vi "Begin.vi"(8 "error in":errorcluster) -> (0 "error out":errorcluster)   [LabVIEW 2014]
doc: "Called before other user functions, this VI is expected to open initial I/O refnums, load in file data, and do all program initialization. Notice that the <B>error out</B> terminal is simply used for data flow. Wiring it to other structures or subVIs ensures that this VI runs first."
uses:
  <vilib>/Rock Robotics/WPI/SafetyOutput/WPI_SafetyOutputConfigMenu.ctl
  <vilib>/Rock Robotics/WPI/DriverStation/WPI_DriverStationRobotMode2.ctl
  <vilib>/Rock Robotics/WPI/Joystick/WPI_JoystickDeviceEnum.ctl
  <vilib>/Rock Robotics/SystemInterfaces/DIO/FPGA_DIOPWMChannel.ctl
  <vilib>/Rock Robotics/SystemInterfaces/spilib/spi_bus.ctl
  <vilib>/Rock Robotics/SystemInterfaces/AI/FPGA_AIGyroChannel.ctl
  <vilib>/Rock Robotics/SystemInterfaces/DIO/FPGA_DIOChannel.ctl
  <vilib>/Rock Robotics/WPI/Encoder/WPI_EncoderType.ctl
  <vilib>/Rock Robotics/WPI/Solenoid/WPI_SolenoidChannel.ctl
  Robot Global Data.vi
  <vilib>/Rock Robotics/Network Tables/SD Write String Array.vi
  <vilib>/Rock Robotics/WPI/RobotDrive/WPI_RobotDriveOpen4MotorWithTalon.vi
  <vilib>/Rock Robotics/WPI/MotorControl/WPI_MotorControlOpen Talon.vi
  <vilib>/Rock Robotics/WPI/Counter/WPI_CounterDigitalInputToDigitalSource.vi
  <vilib>/Rock Robotics/WPI/Compressor/WPI_CompressorGetSetRefNum.vi
  <vilib>/Rock Robotics/WPI/Solenoid/WPI_SolenoidOpenDouble.vi
  NavX/navX-MXP Library/navX-MXP IMU.lvlib
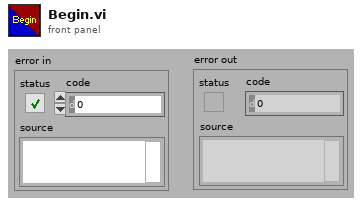
[diagram p1: front panel]
types:
  T1 = typedef "WPI_SolenoidChannel.ctl" = enum8{"Solenoid 0", "Solenoid 1", "Solenoid 2", "Solenoid 3", "Solenoid 4", "Solenoid 5", "Solenoid 6", "Solenoid 7", "Invalid"}
  T2 = typedef "WPI_JoystickDeviceEnum.ctl" = enum16{"USB 0", "USB 1", "USB 2", "USB 3", "USB 4", "USB 5"}
  T3 = typedef "WPI_EncoderType.ctl" = enum16{"1x", "2x", "4x"}
  T4 = typedef "FPGA_DIOPWMChannel.ctl" = enum8{"PWM 0", "PWM 1", "PWM 2", "PWM 3", "PWM 4", "PWM 5", "PWM 6", "PWM 7", "PWM 8", "PWM 9", "PWM MXP 0", "PWM MXP 1", "PWM MXP 2", "PWM MXP 3", "PWM MXP 4", "PWM MXP 5", "PWM MXP 6", "PWM MXP 7", "PWM MXP 8", "PWM MXP 9", "Invalid"}
  T5 = typedef "FPGA_DIOChannel.ctl" = enum8{"DIO 0", "DIO 1", "DIO 2", "DIO 3", "DIO 4", "DIO 5", "DIO 6", "DIO 7", "DIO 8", "DIO 9", "DIO MXP 0", "DIO MXP 1", "DIO MXP 2", "DIO MXP 3", "DIO MXP 4", "DIO MXP 5", "DIO MXP 6", "DIO MXP 7", "DIO MXP 8", "DIO MXP 9", "DIO MXP 10", "DIO MXP 11", "DIO MXP 12", "DIO MXP 13", "DIO MXP 14", "DIO MXP 15", "Invalid"}
  T6 = typedef "FPGA_AIGyroChannel.ctl" = enum8{"AI 0", "AI 1", "Invalid"}
  T7 = typedef "spi_bus.ctl" = enum16{"SPI On-Board, CS0", "SPI On-Board, CS1", "SPI On-Board, CS2", "SPI On-Board, CS3", "SPI MXP", "Invalid"}
  T8 = typedef "WPI_DriverStationRobotMode2.ctl" = enum16{"Autonomous Disabled", "Autonomous Enabled", "Teleop Disabled", "Teleop Enabled", "Disconnected", "Finish", "Test Disabled", "Test Enabled", "Emergency Stopped"}
  T9 = typedef "WPI_SafetyOutputConfigMenu.ctl" = enum16{"Enable", "Disable"}
  T10 = typedef "navX-MXP IMU.lvlib/navX SPI DevRef.ctl" = cluster{"SPIDevRef":T11, "Board Information":T13, "Status":T14, "Offsets":cluster{"Yaw":dbl, "Quat W":dbl, "Quat X":dbl, "Quat Y":dbl, "Quat Z":dbl}, "Update Rate (4Hz-60Hz)":u8, "refnum name":string, "error":errorcluster}
  T11 = typedef "WPI_SPIDevRef.ctl" = cluster{"DevStatus":errorcluster, "Handle":i32, "Controller":T12, "SPI Bus":T7}
  T12 = typedef "FPGA_TypedefDigitalModule.ctl" = enum16{"Controller 1"}
  T13 = typedef "navX-MXP IMU.lvlib/navX Board Information.ctl" = cluster{"WhoAmI (50 | 0x32)":u8, "Board Revision":u8, "Firmware Major Version":u8, "Firmware Minor Version":u8}
  T14 = typedef "navX-MXP IMU.lvlib/navX Status Data.ctl" = cluster{"Update Rate Hz":u8, "Accelerometer Full-Scale Range":u8, "Gyro Full-Scale Range":u16, "NAVX_OP_STATUS":T15, "NAVX_CAL_STATUS":T16, "NAVX_SELFTEST_STATUS":u8, "NAVX_SENSOR_STATUS":T17}
  T15 = typedef "navX-MXP IMU.lvlib/navX NAVX_OP_STATUS.ctl" = u8
  T16 = typedef "navX-MXP IMU.lvlib/navX NAVX_CAL_STATUS.ctl" = u8
  T17 = typedef "navX-MXP IMU.lvlib/navX NAVX_SENSOR_STATUS.ctl" = cluster{"MOVING":bool, "YAW_STABLE":bool, "MAG_DISTURBANCE":bool, "ALTITUDE_VALID":bool, "SEALEVEL_PRESS_SET":bool, "FUSED_HEADING_VALID":bool}
  T18 = cluster{"proportional gain (Kc)":dbl, "integral time (Ti, min)":dbl, "derivative time (Td, min)":dbl}
  T19 = typedef "WPI_DigitalInputDevRef.ctl" = cluster{"DevStatus":errorcluster, "DIO Channel":T5, "Controller":T12}
  T20 = typedef "WPI_GyroDevRef.ctl" = cluster{"DevStatus":errorcluster, "Analog Module":T21, "Analog Channel":T22, "Offset":dbl, "Gain (VoltsPerDegree/Second)":dbl}
  T21 = typedef "FPGA_TypedefAnalogModule.ctl" = enum16{"Controller 1"}
  T22 = typedef "FPGA_AIChannel.ctl" = enum8{"AI 0", "AI 1", "AI 2", "AI 3", "AI MXP 0", "AI MXP 1", "AI MXP 2", "AI MXP 3", "Invalid"}
  T23 = typedef "WPI_JoystickDevRef.ctl" = cluster{"Device":T2}
  T24 = typedef "WPI_CompressorDevRef.ctl" = cluster{"DevStatus":errorcluster, "Pneumatics Control Module":u8}
  T25 = typedef "WPI_MotorControlDeviceRef.ctl" = cluster{"DeviceStatus":errorcluster, "Type":T26, "PWM":cluster{"Controller":T12, "PWM Channel":T4, "DeadBand":T27}, "CAN":cluster{"Device Number":u8, "Control Mode":T28, "Semaphore":T29, "Max Vout":dbl, "TalonSRX Control Mode":T30}, "Invert":bool, "TransformRef":T31, "InvTransformRef":T31}
  T26 = typedef "WPI_MotorControlType.ctl" = enum16{"PWM", "CAN", "CANTalonSRX"}
  T27 = typedef "WPI_PWMDeadband.ctl" = cluster{"Name":string, "maxPositivePwm":i32, "minPositivePwm":i32, "centerPwm":i32, "maxNegativePwm":i32, "minNegativePwm":i32, "angularRange":u16}
  T28 = typedef "WPI_CANJaguar_ControlMode.ctl" = enum8{"Percent VBus", "Current", "Speed", "Position", "Voltage"}
  T29 = typedef "Semaphore RefNum" = refnum<k1>
  T30 = typedef "WPI_CANTalonSRX_APIControlMode.ctl" = enum8{"Percent VBus", "Speed", "Position", "Slave", "Unchanged / Invalid"}
  T31 = typedef "WPI_PWMTransform_ConPane.ctl" = refnum<vi>
  T32 = typedef "WPI_SolenoidDevRef.ctl" = cluster{"DevStatus":errorcluster, "Pneumatics Control Module":u8, "Forward Solenoid Channel":T1, "Reverse Solenoid Channel":T1}
  T33 = typedef "WPI_RobotDriveDevRef.ctl" = cluster{"DevStatus":errorcluster, "Motors[]":T25[], "Square Inputs":bool, "Max Output":dbl}
  T34 = typedef "FPGA_CounterEncoderSourceConvertionLVSourceType.ctl" = cluster{"DevStatus":errorcluster, "AnalogTriggerMode?":bool, "DigitalMode":cluster{"Controller":T12, "DIO Channel":T35}, "AnalogTriggerMode":cluster{"AnalogTriggerIndex":T36, "OutputType":T37}}
  T35 = typedef "FPGA_DIODigitalSourceChannel.ctl" = enum8{"DIO 0", "DIO 1", "DIO 2", "DIO 3", "DIO 4", "DIO 5", "DIO 6", "DIO 7", "DIO 8", "DIO 9", "DIO MXP 0", "DIO MXP 1", "DIO MXP 2", "DIO MXP 3", "DIO MXP 4", "DIO MXP 5", "DIO MXP 6", "DIO MXP 7", "DIO MXP 8", "DIO MXP 9", "DIO MXP 10", "DIO MXP 11", "DIO MXP 12", "DIO MXP 13", "DIO MXP 14", "DIO MXP 15", "Disabled"}
  T36 = typedef "FPGA_AnalogTriggerIndex.ctl" = enum8{"Trig 0", "Trig 1", "Trig 2", "Trig 3", "Trig 4", "Trig 5", "Trig 6", "Trig 7", "Invalid"}
  T37 = typedef "FPGA_AnalogTriggerOutType.ctl" = enum16{"InWindow", "TriggerState", "Rising", "Falling"}
  T38 = typedef "WPI_EncoderDevRef.ctl" = cluster{"DevStatus":errorcluster, "EncoderIndex":T39, "CounterIndex":T40, "DistancePerCount":dbl, "Decoding Type":T3}
  T39 = typedef "FPGA_EncoderIdx.ctl" = enum8{"Enc 0", "Enc 1", "Enc 2", "Enc 3", "Enc 4", "Enc 5", "Enc 6", "Enc 7", "Invalid"}
  T40 = typedef "FPGA_CounterCtrSystemIndex.ctl" = enum8{"Ctr 0", "Ctr 1", "Ctr 2", "Ctr 3", "Ctr 4", "Ctr 5", "Ctr 6", "Ctr 7", "Invalid"}
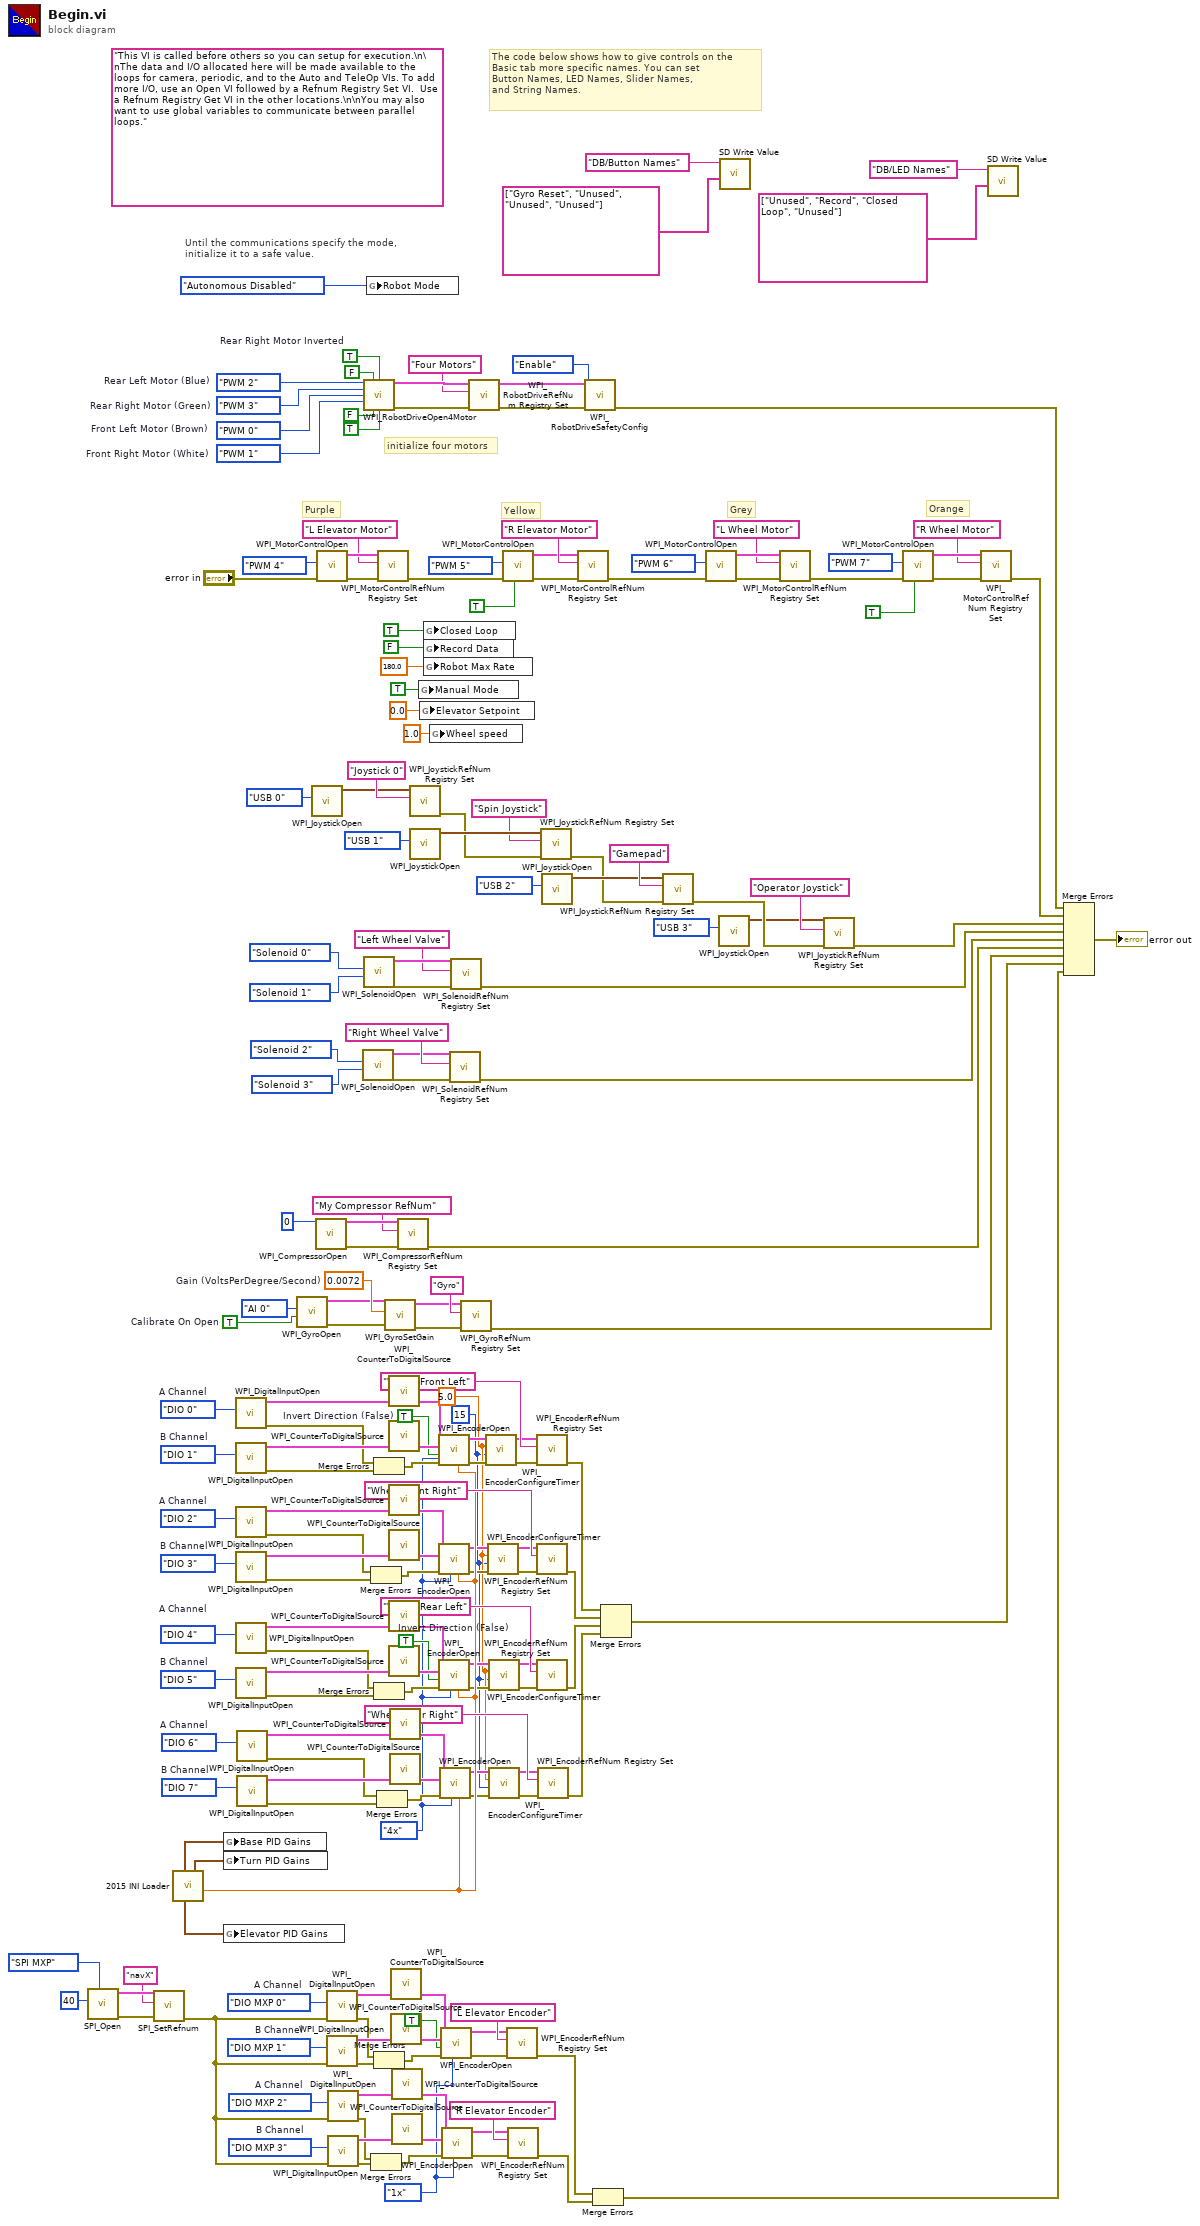
[diagram p0: block diagram]
diagram:
  w22 = u8 15 ("Number Samples to Average")
  w23 = 5.0 ("Minimum Rate")
  w40 = TRUE  # Calibrate On Open
  w19 = WPI_EncoderType."1x" ("Decoding Type")
  w52 = WPI_EncoderType."4x" ("Decoding Type")
  w53 = TRUE  # Invert Direction (False)
  w54 = TRUE  # Invert Direction (False)
  w122 = FPGA_DIOChannel."DIO MXP 3"  # B Channel
  w121 = FPGA_DIOChannel."DIO MXP 2"  # A Channel
  w107 = FPGA_DIOChannel."DIO MXP 1"  # B Channel
  w108 = FPGA_DIOChannel."DIO MXP 0"  # A Channel
  w133 = FPGA_DIOChannel."DIO 7"  # B Channel
  w134 = FPGA_DIOChannel."DIO 6"  # A Channel
  w144 = FPGA_DIOChannel."DIO 5"  # B Channel
  w143 = FPGA_DIOChannel."DIO 4"  # A Channel
  w145 = FPGA_DIOChannel."DIO 3"  # B Channel
  w146 = FPGA_DIOChannel."DIO 2"  # A Channel
  w156 = FPGA_DIOChannel."DIO 1"  # B Channel
  w155 = FPGA_DIOChannel."DIO 0"  # A Channel
  w165 = 0.0072  # Gain (VoltsPerDegree/Second)
  w180 = TRUE  # Rear Right Motor Inverted
  w185 = FPGA_DIOPWMChannel."PWM 1"  # Front Right Motor (White)
  w186 = FPGA_DIOPWMChannel."PWM 0"  # Front Left Motor (Brown)
  w187 = FPGA_DIOPWMChannel."PWM 3"  # Rear Right Motor (Green)
  w188 = FPGA_DIOPWMChannel."PWM 2"  # Rear Left Motor (Blue)
  (unwired) "This VI is called before others so you can setup for execution.\n\nThe data and I/O allocated here will be made available to the loops for camera, periodic, and to the Auto and TeleOp VIs. To add more I/O, use an Open VI followed by a Refnum Registry Set VI.  Use a Refnum Registry Get VI in the other locations.\n\nYou may also want to use global variables to communicate between parallel loops."
  # "Orange"
  # "Grey"
  # "Purple"
  # "Yellow"
  # "The code below shows how to give controls on the\nBasic tab more specific names. You can set\nButton Names, LED Names, Slider Names,\nand String Names."
  # "Until the communications specify the mode,\ninitialize it to a safe value."
  # "initialize four motors"
  n1 = call "SPI_Open.vi"("SPI Bus (SPI MXP)"=spi_bus."SPI MXP", "Update Rate (4Hz-60Hz)"=u8 40) -> ("error out"=w171:errorcluster, "navX DevRef"=w172:T10)  [unwired: 7 in, 1 out]
  n2 = call "SPI_SetRefnum.vi"("error in (no error)"=w171, "refnum name"="navX", "navX DevRef"=w172) -> ("error out"=w55:errorcluster)  [unwired: 7 in, 1 out]
  n3 = call "2015 INI Loader.vi"() -> ("Inches Per Tick"=w51:dbl, "Turn PID gains"=w48:T18, "Elevator PID gains"=w49:T18, "Base PID gains"=w50:T18)  [unwired: 6 in, 2 out]
  n4 = global write "Robot Global Data.vi" "Base PID Gains"(w50) -> ()
  n5 = global write "Robot Global Data.vi" "Turn PID Gains"(w48) -> ()
  n6 = global write "Robot Global Data.vi" "Elevator PID Gains"(w49) -> ()
  n7 = call <vilib>:"WPI_DigitalInputOpen.vi"("DIO Channel"=w155) -> ("error out"=w81:errorcluster, "DigitalInputDevRef"=w152:T19)  [unwired: 2 in, 7 out]
  n8 = call <vilib>:"WPI_DigitalInputOpen.vi"("DIO Channel"=w156) -> ("error out"=w82:errorcluster, "DigitalInputDevRef"=w153:T19)  [unwired: 2 in, 7 out]
  n9 = call <vilib>:"WPI_DigitalInputOpen.vi"("DIO Channel"=w146) -> ("error out"=w73:errorcluster, "DigitalInputDevRef"=w149:T19)  [unwired: 2 in, 7 out]
  n10 = call <vilib>:"WPI_DigitalInputOpen.vi"("DIO Channel"=w145) -> ("error out"=w76:errorcluster, "DigitalInputDevRef"=w148:T19)  [unwired: 2 in, 7 out]
  n11 = call <vilib>:"WPI_DigitalInputOpen.vi"("DIO Channel"=w143) -> ("error out"=w77:errorcluster, "DigitalInputDevRef"=w140:T19)  [unwired: 2 in, 7 out]
  n12 = call <vilib>:"WPI_DigitalInputOpen.vi"("DIO Channel"=w144) -> ("error out"=w78:errorcluster, "DigitalInputDevRef"=w141:T19)  [unwired: 2 in, 7 out]
  n13 = call <vilib>:"WPI_DigitalInputOpen.vi"("DIO Channel"=w134) -> ("error out"=w71:errorcluster, "DigitalInputDevRef"=w137:T19)  [unwired: 2 in, 7 out]
  n14 = call <vilib>:"WPI_DigitalInputOpen.vi"("DIO Channel"=w133) -> ("error out"=w72:errorcluster, "DigitalInputDevRef"=w136:T19)  [unwired: 2 in, 7 out]
  n15 = call <vilib>:"WPI_GyroOpen.vi"("Calibrate On Open"=w40, "Analog Channel"=FPGA_AIGyroChannel."AI 0") -> ("error out"=w162:errorcluster, "GyroDevRef"=w164:T20)  [unwired: 7 in, 1 out]
  n16 = call <vilib>:"WPI_JoystickOpen.vi"("JoystickDevice"=WPI_JoystickDeviceEnum."USB 0") -> ("JoystickDevRef"=w190:T23)  [unwired: 10 in]
  n17 = call <vilib>:"WPI_CompressorOpen.vi"("Pneumatics Control Module (0)"=u8 0) -> ("CompressorDevRef"=w128:T24, "error out"=w127:errorcluster)  [unwired: 13 in]
  n18 = call-poly <vilib>:"WPI_MotorControlOpen.vi"("error in (no error)"="error in", "PWM Channel"=FPGA_DIOPWMChannel."PWM 4") -> ("error out"=w97:errorcluster, "MotorControlDeviceRef"=w159:T25)  [unwired: 8 in]
  n19 = call <vilib>:"WPI_DigitalInputOpen.vi"("error in (no error)"=w55, "DIO Channel"=w108) -> ("error out"=w62:errorcluster, "DigitalInputDevRef"=w111:T19)  [unwired: 1 in, 7 out]
  n20 = call <vilib>:"WPI_DigitalInputOpen.vi"("error in (no error)"=w55, "DIO Channel"=w107) -> ("error out"=w65:errorcluster, "DigitalInputDevRef"=w110:T19)  [unwired: 1 in, 7 out]
  n21 = call <vilib>:"WPI_DigitalInputOpen.vi"("error in (no error)"=w55, "DIO Channel"=w121) -> ("error out"=w63:errorcluster, "DigitalInputDevRef"=w118:T19)  [unwired: 1 in, 7 out]
  n22 = call <vilib>:"WPI_DigitalInputOpen.vi"("error in (no error)"=w55, "DIO Channel"=w122) -> ("error out"=w64:errorcluster, "DigitalInputDevRef"=w119:T19)  [unwired: 1 in, 7 out]
  n23 = call-poly <vilib>:"WPI_SolenoidOpen.vi"("Reverse Solenoid Channel"=WPI_SolenoidChannel."Solenoid 3", "Forward Solenoid Channel"=WPI_SolenoidChannel."Solenoid 2") -> ("error out"=w13:errorcluster, "SolenoidDevRef"=w11:T32)  [unwired: 8 in]
  n24 = call-poly <vilib>:"WPI_RobotDriveOpen4Motor.vi"("Rear Left Motor"=w188, "Rear Left Motor Inverted"=FALSE, "Rear Right Motor Inverted"=w180, "Rear Right Motor"=w187, "Front Left Motor"=w186, "Front Right Motor"=w185, "Front Left Motor Inverted"=FALSE, "Front Right Motor Inverted"=TRUE) -> ("RobotDriveDevRef"=w197:T33, "error out"=w195:errorcluster)  [unwired: 6 in]
  n25 = call-poly <vilib>:"WPI_SolenoidOpen.vi"("Reverse Solenoid Channel"=WPI_SolenoidChannel."Solenoid 1", "Forward Solenoid Channel"=WPI_SolenoidChannel."Solenoid 0") -> ("error out"=w14:errorcluster, "SolenoidDevRef"=w16:T32)  [unwired: 8 in]
  n26 = global write "Robot Global Data.vi" "Robot Mode"(WPI_DriverStationRobotMode2."Autonomous Disabled" ("Robot Mode")) -> ()
  n27 = Merge Errors(w73, w76) -> (w75:errorcluster)
  n28 = Merge Errors(w63, w64) -> (w61:errorcluster)
  n29 = Merge Errors(w81, w82) -> (w80:errorcluster)
  n30 = Merge Errors(w77, w78) -> (w74:errorcluster)
  n31 = Merge Errors(w62, w65) -> (w60:errorcluster)
  n32 = Merge Errors(w71, w72) -> (w79:errorcluster)
  n33 = call <vilib>:"WPI_MotorControlRefNum Registry Set.vi"("error in (no error)"=w97, "refnum name"="L Elevator Motor", "MotorControlDevRef"=w159) -> ("error out"=w96:errorcluster)  [unwired: 7 in, 1 out]
  n34 = call <vilib>:"WPI_GyroSetGain.vi"("error in (no error)"=w162, "Gain (VoltsPerDegree/Second)"=w165, "GyroDevRef"=w164) -> ("error out"=w161:errorcluster, "GyroDevRef"=w163:T20)  [unwired: 7 in]
  n35 = call-poly <vilib>:"WPI_CounterToDigitalSource.vi"("DigitalInputDevRef"=w152) -> ("Digital Source"=w151:T34)  [unwired: 6 out]
  n36 = call-poly <vilib>:"WPI_CounterToDigitalSource.vi"("DigitalInputDevRef"=w153) -> ("Digital Source"=w154:T34)  [unwired: 6 out]
  n37 = call-poly <vilib>:"WPI_CounterToDigitalSource.vi"("DigitalInputDevRef"=w149) -> ("Digital Source"=w150:T34)  [unwired: 6 out]
  n38 = call-poly <vilib>:"WPI_CounterToDigitalSource.vi"("DigitalInputDevRef"=w148) -> ("Digital Source"=w147:T34)  [unwired: 6 out]
  n39 = call-poly <vilib>:"WPI_CounterToDigitalSource.vi"("DigitalInputDevRef"=w140) -> ("Digital Source"=w139:T34)  [unwired: 6 out]
  n40 = call-poly <vilib>:"WPI_CounterToDigitalSource.vi"("DigitalInputDevRef"=w141) -> ("Digital Source"=w142:T34)  [unwired: 6 out]
  n41 = call-poly <vilib>:"WPI_CounterToDigitalSource.vi"("DigitalInputDevRef"=w137) -> ("Digital Source"=w138:T34)  [unwired: 6 out]
  n42 = call-poly <vilib>:"WPI_CounterToDigitalSource.vi"("DigitalInputDevRef"=w136) -> ("Digital Source"=w135:T34)  [unwired: 6 out]
  n43 = call-poly <vilib>:"WPI_CounterToDigitalSource.vi"("DigitalInputDevRef"=w111) -> ("Digital Source"=w112:T34)  [unwired: 6 out]
  n44 = call-poly <vilib>:"WPI_CounterToDigitalSource.vi"("DigitalInputDevRef"=w110) -> ("Digital Source"=w109:T34)  [unwired: 6 out]
  n45 = call-poly <vilib>:"WPI_CounterToDigitalSource.vi"("DigitalInputDevRef"=w118) -> ("Digital Source"=w117:T34)  [unwired: 6 out]
  n46 = call-poly <vilib>:"WPI_CounterToDigitalSource.vi"("DigitalInputDevRef"=w119) -> ("Digital Source"=w120:T34)  [unwired: 6 out]
  n47 = call <vilib>:"WPI_CompressorRefNum Registry Set.vi"("error in (no error)"=w127, "refnum name"="My Compressor RefNum", "CompressorDevRef"=w128) -> ("error out"=w84:errorcluster)  [unwired: 7 in, 1 out]
  n48 = call <vilib>:"WPI_JoystickRefNum Registry Set.vi"("refnum name"="Joystick 0", "JoystickDevRef"=w190) -> ("error out"=w86:errorcluster)  [unwired: 8 in, 1 out]
  n49 = call <vilib>:"WPI_JoystickOpen.vi"("JoystickDevice"=WPI_JoystickDeviceEnum."USB 1") -> ("JoystickDevRef"=w177:T23)  [unwired: 10 in]
  n50 = global write "Robot Global Data.vi" "Manual Mode"(TRUE ("Manual Mode")) -> ()
  n51 = global write "Robot Global Data.vi" "Elevator Setpoint"(0.0 ("Robot Max Rate")) -> ()
  n52 = global write "Robot Global Data.vi" "Closed Loop"(TRUE ("Closed Loop")) -> ()
  n53 = global write "Robot Global Data.vi" "Record Data"(FALSE ("Enable Vision")) -> ()
  n54 = global write "Robot Global Data.vi" "Robot Max Rate"(180.0 ("Robot Max Rate")) -> ()
  n55 = global write "Robot Global Data.vi" "Wheel speed"(1.0 ("Wheel speed")) -> ()
  n56 = call <vilib>:"WPI_EncoderOpen.vi"("DistancePerCount"=w51, "Decoding Type"=w52, "error in (no error)"=w80, "Invert Direction (False)"=w53, "BSource"=w154, "ASource"=w151) -> ("error out"=w38:errorcluster, "EncoderDevRef"=w39:T38)  [unwired: 2 in, 2 out]
  n57 = call <vilib>:"WPI_EncoderOpen.vi"("DistancePerCount"=w51, "Decoding Type"=w52, "error in (no error)"=w75, "BSource"=w147, "ASource"=w150) -> ("error out"=w34:errorcluster, "EncoderDevRef"=w35:T38)  [unwired: 3 in, 2 out]
  n58 = call <vilib>:"WPI_EncoderOpen.vi"("DistancePerCount"=w51, "Decoding Type"=w52, "error in (no error)"=w74, "Invert Direction (False)"=w54, "BSource"=w142, "ASource"=w139) -> ("error out"=w30:errorcluster, "EncoderDevRef"=w31:T38)  [unwired: 2 in, 2 out]
  n59 = call <vilib>:"WPI_EncoderOpen.vi"("DistancePerCount"=w51, "Decoding Type"=w52, "error in (no error)"=w79, "BSource"=w135, "ASource"=w138) -> ("error out"=w26:errorcluster, "EncoderDevRef"=w27:T38)  [unwired: 3 in, 2 out]
  n60 = call <vilib>:"WPI_EncoderOpen.vi"("Decoding Type"=w19, "error in (no error)"=w60, "Invert Direction (False)"=TRUE, "BSource"=w109, "ASource"=w112) -> ("error out"=w113:errorcluster, "EncoderDevRef"=w114:T38)  [unwired: 3 in, 2 out]
  n61 = call <vilib>:"WPI_EncoderOpen.vi"("Decoding Type"=w19, "error in (no error)"=w61, "BSource"=w120, "ASource"=w117) -> ("error out"=w116:errorcluster, "EncoderDevRef"=w115:T38)  [unwired: 4 in, 2 out]
  n62 = call <vilib>:"WPI_SolenoidRefNum Registry Set.vi"("error in (no error)"=w13, "refnum name"="Right Wheel Valve", "SolenoidDevRef"=w11) -> ("error out"=w5:errorcluster)  [unwired: 7 in, 1 out]
  n63 = call <vilib>:"WPI_SolenoidRefNum Registry Set.vi"("error in (no error)"=w14, "refnum name"="Left Wheel Valve", "SolenoidDevRef"=w16) -> ("error out"=w6:errorcluster)  [unwired: 7 in, 1 out]
  n64 = call <vilib>:"WPI_GyroRefNum Registry Set.vi"("error in (no error)"=w161, "refnum name"="Gyro", "GyroDevRef"=w163) -> ("error out"=w83:errorcluster)  [unwired: 7 in, 1 out]
  n65 = call <vilib>:"WPI_RobotDriveRefNum Registry Set.vi"("error in (no error)"=w195, "refnum name"="Four Motors", "RobotDriveDevRef"=w197) -> ("error out"=w90:errorcluster, "RobotDriveDevRef"=w194:T33)  [unwired: 7 out]
  n66 = call <vilib>:"WPI_EncoderConfigureTimer.vi"("error in (no error)"=w38, "Number Samples to Average"=w22, "Minimum Rate"=w23, "EncoderDevRef"=w39) -> ("error out"=w37:errorcluster, "EncoderDevRef"=w36:T38)  [unwired: 6 in]
  n67 = call <vilib>:"WPI_EncoderConfigureTimer.vi"("error in (no error)"=w34, "Number Samples to Average"=w22, "Minimum Rate"=w23, "EncoderDevRef"=w35) -> ("error out"=w33:errorcluster, "EncoderDevRef"=w32:T38)  [unwired: 6 in]
  n68 = call <vilib>:"WPI_EncoderConfigureTimer.vi"("error in (no error)"=w30, "Number Samples to Average"=w22, "Minimum Rate"=w23, "EncoderDevRef"=w31) -> ("error out"=w29:errorcluster, "EncoderDevRef"=w28:T38)  [unwired: 6 in]
  n69 = call <vilib>:"WPI_EncoderConfigureTimer.vi"("error in (no error)"=w26, "Number Samples to Average"=w22, "Minimum Rate"=w23, "EncoderDevRef"=w27) -> ("error out"=w25:errorcluster, "EncoderDevRef"=w24:T38)  [unwired: 6 in]
  n70 = call-poly <vilib>:"WPI_MotorControlOpen.vi"("Invert"=TRUE, "error in (no error)"=w96, "PWM Channel"=FPGA_DIOPWMChannel."PWM 5") -> ("error out"=w95:errorcluster, "MotorControlDeviceRef"=w105:T25)  [unwired: 7 in]
  n71 = call <vilib>:"WPI_EncoderRefNum Registry Set.vi"("error in (no error)"=w113, "refnum name"="L Elevator Encoder", "EncoderDevRef"=w114) -> ("error out"=w59:errorcluster)  [unwired: 7 in, 1 out]
  n72 = call <vilib>:"WPI_EncoderRefNum Registry Set.vi"("error in (no error)"=w116, "refnum name"="R Elevator Encoder", "EncoderDevRef"=w115) -> ("error out"=w58:errorcluster)  [unwired: 7 in, 1 out]
  n73 = call <vilib>:"WPI_EncoderRefNum Registry Set.vi"("error in (no error)"=w37, "refnum name"="Wheel Front Left", "EncoderDevRef"=w36) -> ("error out"=w70:errorcluster)  [unwired: 7 in, 1 out]
  n74 = call <vilib>:"WPI_EncoderRefNum Registry Set.vi"("error in (no error)"=w33, "refnum name"="Wheel Front Right", "EncoderDevRef"=w32) -> ("error out"=w69:errorcluster)  [unwired: 7 in, 1 out]
  n75 = call <vilib>:"WPI_EncoderRefNum Registry Set.vi"("error in (no error)"=w29, "refnum name"="Wheel Rear Left", "EncoderDevRef"=w28) -> ("error out"=w68:errorcluster)  [unwired: 7 in, 1 out]
  n76 = call <vilib>:"WPI_EncoderRefNum Registry Set.vi"("error in (no error)"=w25, "refnum name"="Wheel Rear Right", "EncoderDevRef"=w24) -> ("error out"=w67:errorcluster)  [unwired: 7 in, 1 out]
  n77 = call <vilib>:"WPI_JoystickRefNum Registry Set.vi"("error in (no error)"=w86, "refnum name"="Spin Joystick", "JoystickDevRef"=w177) -> ("error out"=w85:errorcluster)  [unwired: 7 in, 1 out]
  n78 = call <vilib>:"WPI_JoystickOpen.vi"("JoystickDevice"=WPI_JoystickDeviceEnum."USB 2") -> ("JoystickDevRef"=w174:T23)  [unwired: 10 in]
  n79 = call <vilib>:"WPI_MotorControlRefNum Registry Set.vi"("error in (no error)"=w95, "refnum name"="R Elevator Motor", "MotorControlDevRef"=w105) -> ("error out"=w94:errorcluster)  [unwired: 7 in, 1 out]
  n80 = call <vilib>:"WPI_RobotDriveSafetyConfig.vi"("error in (no error)"=w90, "mode"=WPI_SafetyOutputConfigMenu."Enable", "RobotDriveDevRef"=w194) -> ("error out"=w56:errorcluster)  [unwired: 7 in, 1 out]
  n81 = Merge Errors(w59, w58) -> (w57:errorcluster)
  n82 = Merge Errors(w70, w69, w68, w67) -> (w66:errorcluster)
  n83 = call <vilib>:"WPI_JoystickRefNum Registry Set.vi"("error in (no error)"=w85, "refnum name"="Gamepad", "JoystickDevRef"=w174) -> ("error out"=w44:errorcluster)  [unwired: 7 in, 1 out]
  n84 = call-poly <vilib>:"WPI_MotorControlOpen.vi"("error in (no error)"=w94, "PWM Channel"=FPGA_DIOPWMChannel."PWM 6") -> ("error out"=w93:errorcluster, "MotorControlDeviceRef"=w100:T25)  [unwired: 8 in]
  n85 = call <vilib>:"WPI_JoystickOpen.vi"("JoystickDevice"=WPI_JoystickDeviceEnum."USB 3") -> ("JoystickDevRef"=w41:T23)  [unwired: 10 in]
  n86 = call-poly <vilib>:"SD Write Value.vi"("String Array"=string[] ["Gyro Reset", "Unused", "Unused", "Unused"], "Name"="DB/Button Names") -> ()  [unwired: 8 in, 2 out]
  n87 = call <vilib>:"WPI_MotorControlRefNum Registry Set.vi"("error in (no error)"=w93, "refnum name"="L Wheel Motor", "MotorControlDevRef"=w100) -> ("error out"=w92:errorcluster)  [unwired: 7 in, 1 out]
  n88 = call <vilib>:"WPI_JoystickRefNum Registry Set.vi"("error in (no error)"=w44, "refnum name"="Operator Joystick", "JoystickDevRef"=w41) -> ("error out"=w43:errorcluster)  [unwired: 7 in, 1 out]
  n89 = call-poly <vilib>:"WPI_MotorControlOpen.vi"("Invert"=TRUE, "error in (no error)"=w92, "PWM Channel"=FPGA_DIOPWMChannel."PWM 7") -> ("error out"=w91:errorcluster, "MotorControlDeviceRef"=w102:T25)  [unwired: 7 in]
  n90 = call <vilib>:"WPI_MotorControlRefNum Registry Set.vi"("error in (no error)"=w91, "refnum name"="R Wheel Motor", "MotorControlDevRef"=w102) -> ("error out"=w87:errorcluster)  [unwired: 7 in, 1 out]
  n91 = call-poly <vilib>:"SD Write Value.vi"("String Array"=string[] ["Unused", "Record", "Closed Loop", "Unused"], "Name"="DB/LED Names") -> ()  [unwired: 8 in, 2 out]
  n92 = Merge Errors(w56, w87, w43, w6, w5, w84, w83, w66, w57) -> (→"error out":errorcluster)
